vi "learning_phase.vi"(1 "Weights 2":dbl[][](array[numeric]), 4 "Weights 1":dbl[][](array[numeric]), 5 "Learning Rate":dbl(slide)=0.336734693877551 scale=0.0..1.0, 6 "Beta":dbl(slide)=1.0 scale=0.0..1.0, 7 "inputs":T1) -> (0 "Error":dbl(graph), 2 "Weight_2_out":dbl[][](array[numeric]), 3 "Weight_1_out":dbl[][](array[numeric]))   [LabVIEW 2009]
panel:
  # "Artificial Neural Network Learning"
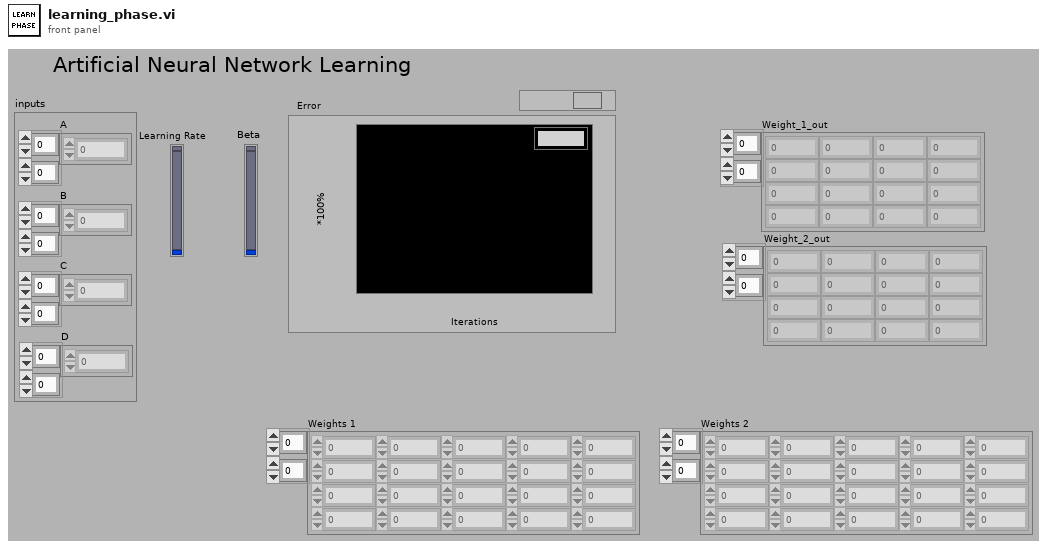
[diagram p1: front panel]
types:
  T1 = cluster{"B":dbl[][], "C":dbl[][], "D":dbl[][], "A":dbl[][]}
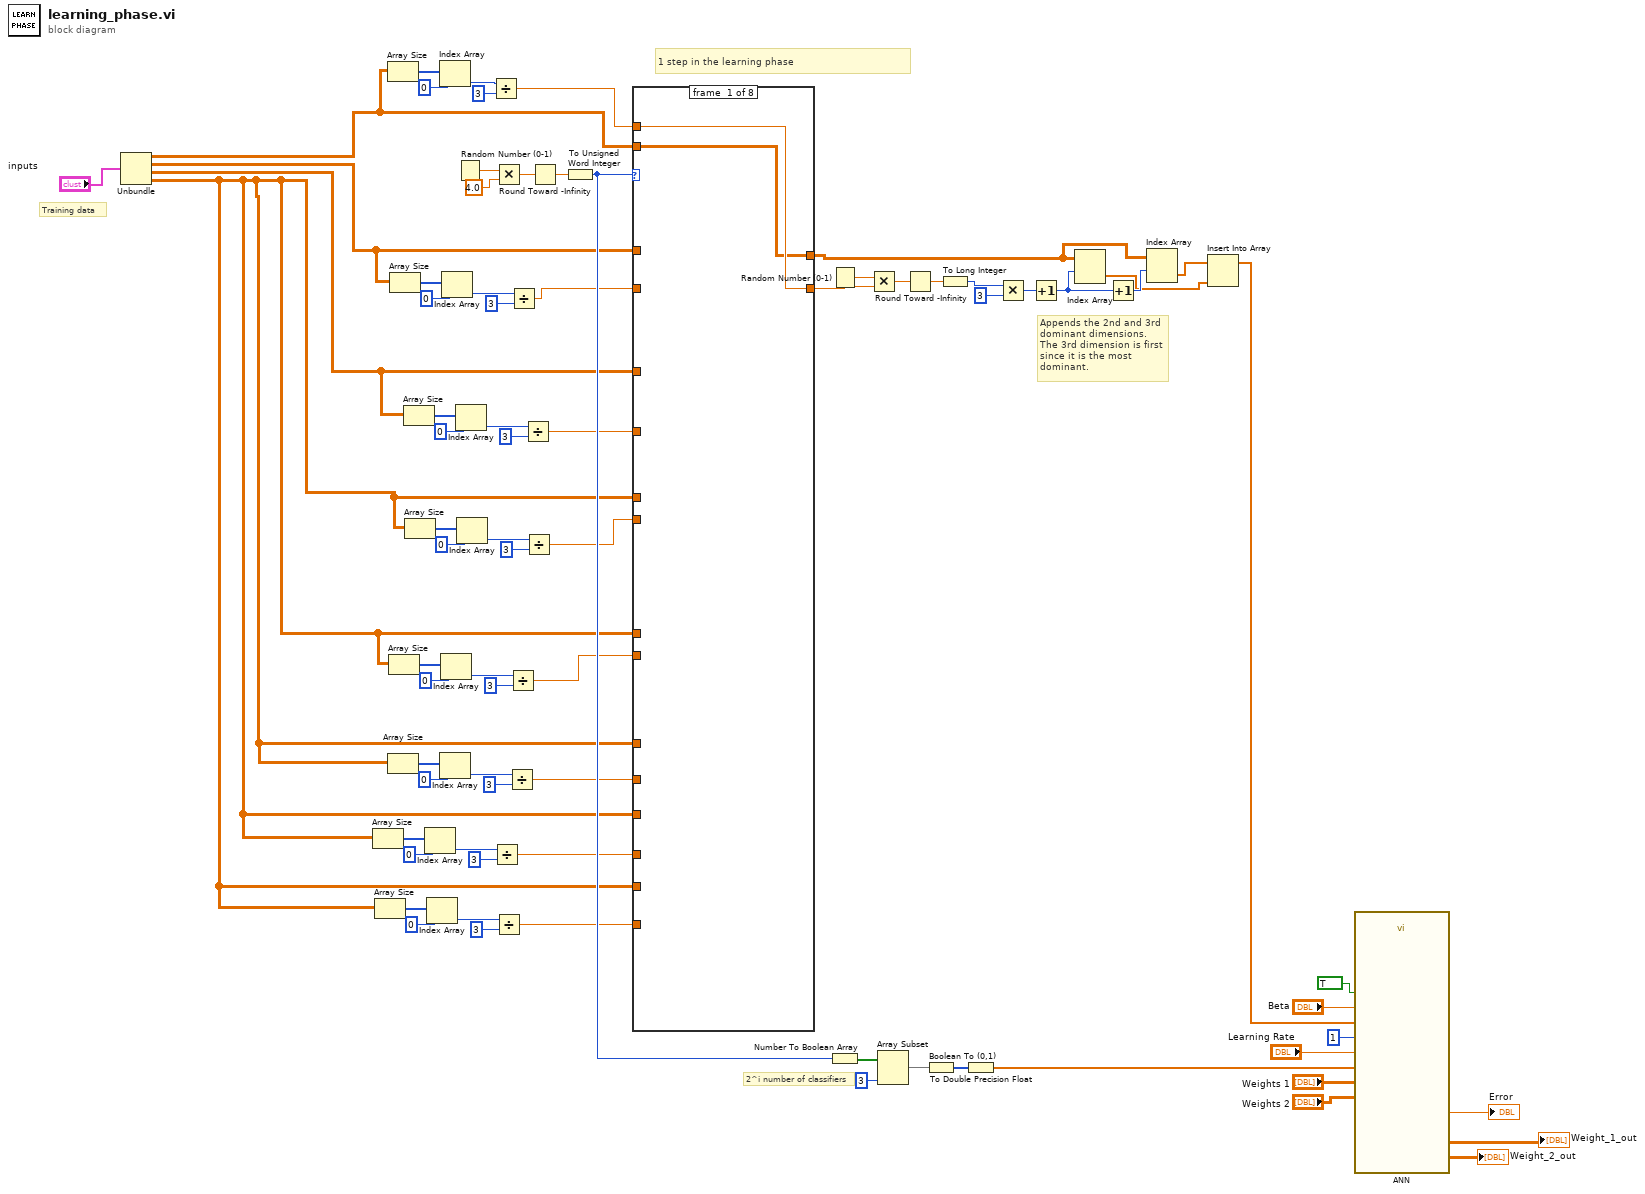
[diagram p0: block diagram]
diagram:
  # "Appends the 2nd and 3rd dominant dimensions. The 3rd dimension is first since it is the most dominant."
  # "2^i number of classifiers"
  # "Training data"
  # "1 step in the learning phase"
  n1 = Unbundle("inputs") -> ("B"=w32:dbl[][], "C"=w30:dbl[][], "D"=w28:dbl[][], "A"=w1:dbl[][])
  n2 = Array Size(array=w1) -> (size(s)=w12:i32[])
  n3 = Array Size(array=w1) -> (size(s)=w8:i32[])
  n4 = Array Size(array=w32) -> (size(s)=w77:i32[])
  n5 = Array Size(array=w1) -> (size(s)=w16:i32[])
  n6 = Array Size(array=w1) -> (size(s)=w22:i32[])
  n7 = Array Size(array=w30) -> (size(s)=w74:i32[])
  n8 = Array Size(array=w28) -> (size(s)=w51:i32[])
  n9 = Array Size(array=w1) -> (size(s)=w47:i32[])
  n10 = Index Array(array=w12, index=0) -> (element=w10:i32)
  n11 = Index Array(array=w8, index=0) -> (element=w6:i32)
  n12 = Index Array(array=w77, index=0) -> (element=w72:i32)
  n13 = Index Array(array=w16, index=0) -> (element=w14:i32)
  n14 = Index Array(array=w22, index=0) -> (element=w20:i32)
  n15 = Index Array(array=w74, index=0) -> (element=w70:i32)
  n16 = Random Number (0-1)() -> (number: 0 to 1=w68:dbl)
  n17 = Index Array(array=w51, index=0) -> (element=w49:i32)
  n18 = Index Array(array=w47, index=0) -> (element=w45:i32)
  n19 = Divide(x=w72, y=3) -> (x/y=w33:dbl)
  n20 = Divide(x=w10, y=3) -> (x/y=w3:dbl)
  n21 = Multiply(x=w68, y=4.0) -> (x*y=w66:dbl)
  n22 = Divide(x=w6, y=3) -> (x/y=w2:dbl)
  n23 = Divide(x=w14, y=3) -> (x/y=w4:dbl)
  n24 = Divide(x=w20, y=3) -> (x/y=w18:dbl)
  n25 = Divide(x=w70, y=3) -> (x/y=w29:dbl)
  n26 = Divide(x=w49, y=3) -> (x/y=w27:dbl)
  n27 = Divide(x=w45, y=3) -> (x/y=w26:dbl)
  n28 = Round Toward -Infinity(1:w66) -> (0:w65:dbl)
  n29 = To Unsigned Word Integer(number=w65) -> (unsigned 16bit integer=w31:u16)
  n30 = case shown="4" w31 {
    tunnel: w33 -> [w79 _ _ _ _ _ _ _]
    tunnel: w32 -> [w78 _ _ _ _ _ _ _]
    tunnel: w30 -> [_ w81 _ _ _ _ _ _]
    tunnel: w29 -> [_ w80 _ _ _ _ _ _]
    tunnel: w28 -> [_ _ w83 _ _ _ _ _]
    tunnel: w27 -> [_ _ w82 _ _ _ _ _]
    tunnel: w1 -> [_ _ _ w85 _ _ _ _]
    tunnel: w26 -> [_ _ _ w84 _ _ _ _]
    tunnel: [w79 w80 w82 w84 w86 w88 w90 w92] -> w25
    tunnel: [w78 w81 w83 w85 w87 w89 w91 w93] -> w24
    tunnel: w1 -> [_ _ _ _ w87 _ _ _]
    tunnel: w18 -> [_ _ _ _ w86 _ _ _]
    tunnel: w1 -> [_ _ _ _ _ w89 _ _]
    tunnel: w1 -> [_ _ _ _ _ _ w91 _]
    tunnel: w1 -> [_ _ _ _ _ _ _ w93]
    tunnel: w4 -> [_ _ _ _ _ w88 _ _]
    tunnel: w3 -> [_ _ _ _ _ _ w90 _]
    tunnel: w2 -> [_ _ _ _ _ _ _ w92]
    frame #0 {
    }
    frame #1 {
    }
    frame #2 {
    }
    frame #3 {
    }
    frame #4 {
    }
    frame #5 {
    }
    frame #6 {
    }
    frame #7 {
    }
  }
  n31 = Random Number (0-1)() -> (number: 0 to 1=w43:dbl)
  n32 = Number To Boolean Array(number=w31) -> (Boolean array=w59:bool[])
  n33 = Multiply(x=w43, y=w25) -> (x*y=w42:dbl)
  n34 = Array Subset(array=w59, length=3) -> (w57:bool[])  [unwired: 1 in]
  n35 = Round Toward -Infinity(1:w42) -> (0:w41:dbl)
  n36 = Boolean To (0,1)(Boolean=w57) -> (0, 1=w56:i16[])
  n37 = To Long Integer(number=w41) -> (32bit integer=w40:i32)
  n38 = To Double Precision Float(number=w56) -> (double precision float=w55:dbl[])
  n39 = Multiply(x=w40, y=3) -> (x*y=w38:i32)
  n40 = Increment(x=w38) -> (x+1=w37:i32)
  n41 = Index Array(array=w24, index (row)=w37) -> (element=w34:dbl[])  [unwired: 1 in]
  n42 = Increment(x=w37) -> (x+1=w36:i32)
  n43 = Index Array(array=w24, index (row)=w36) -> (element=w35:dbl[])  [unwired: 1 in]
  n44 = Insert Into Array(array=w35, new element=w34) -> (w23:dbl[])  [unwired: 1 in]
  n45 = call "ANN.vi"("Input"=w23, "Iterations"=1, "Beta"="Beta", "Target Output"=w55, "Weight_2"="Weights 2", "Weight_1"="Weights 1", "Back Propagation"=TRUE, "Learning Rate"="Learning Rate") -> ("Weight_2_out"=→"Weight_2_out":dbl[][], "Weight_1_out"=→"Weight_1_out":dbl[][], "Error"=→"Error":dbl)  [unwired: 4 in, 1 out]
